vi "04TRM800.vi"() -> ()   [LabVIEW 2015]
uses:
  <vilib>/Utility/error.llb/DialogType.ctl
  <vilib>/Instr/_visa.llb/VISA Configure Serial Port (Serial Instr).vi
panel:
  out "Messages":string
  in  "INC":dbl min=-3.0 max=15.0 step=0.5 format="%.1g"
  in  "stop":bool
  out "String":string
  in  "LPCA COM Port":refnum<visa-resource-name>
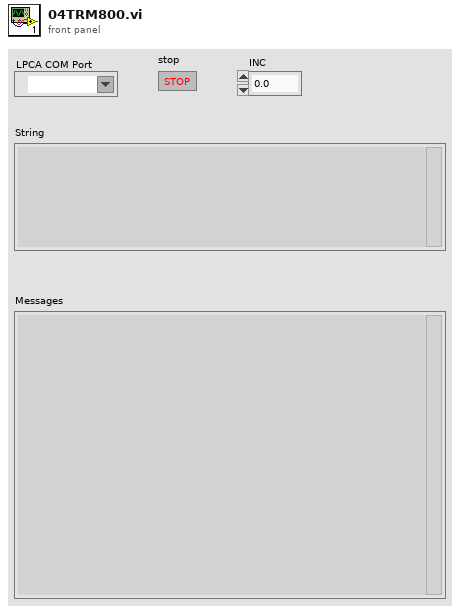
[diagram p1: front panel]
types:
  T1 = enum16{"Initialize", "Error", "Close", "Next", "Send"}
  T2 = enum16{"Initialize", "Next", "SendRSET", "SetMPH", "SetINC"}
  T3 = typedef "DialogType.ctl" = u16
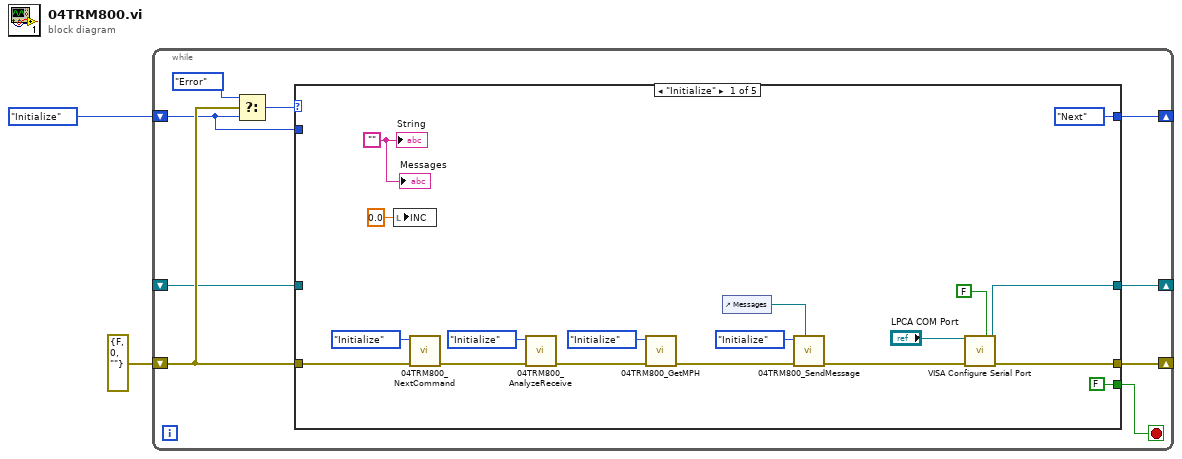
[diagram p0: block diagram]
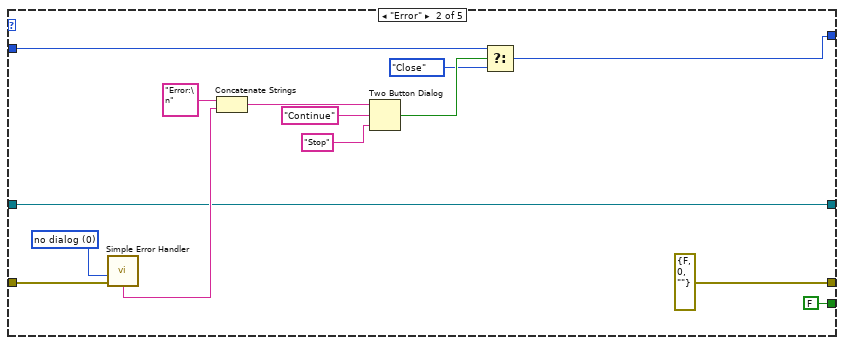
[diagram p2: hidden frame]
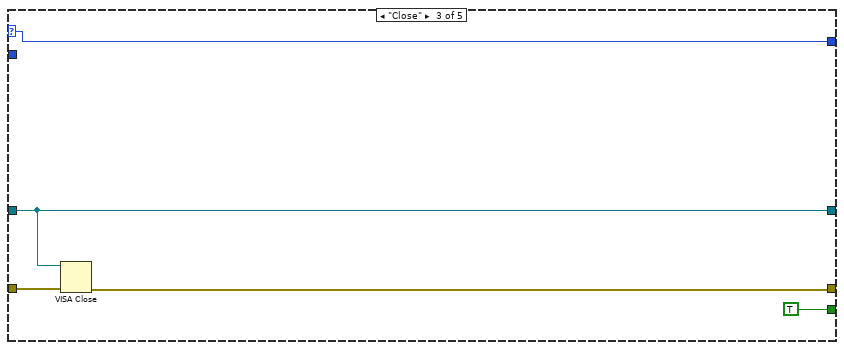
[diagram p3: hidden frame]
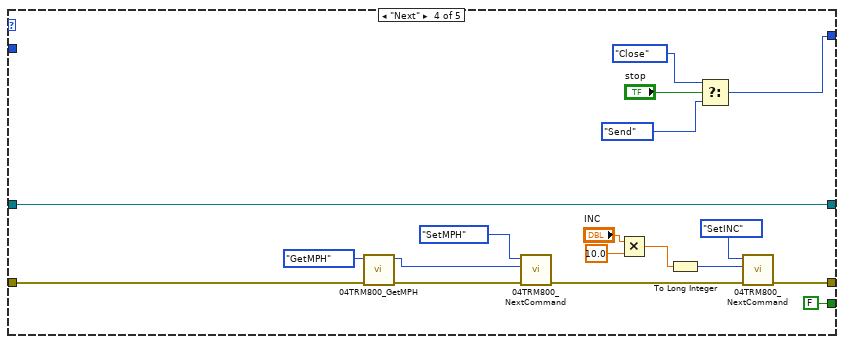
[diagram p4: hidden frame]
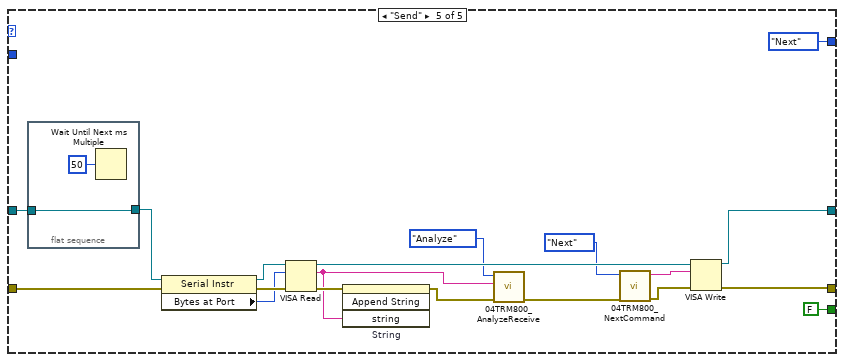
[diagram p5: hidden frame]
diagram:
  n1 = while {
    shift-right: [w9] -> _
    shift-left: T1."Initialize" -> [w8]
    shift-right: [w7] -> _
    shift-left: errorcluster {"status"=FALSE, "code"=0, "source"=""} ("error constant") -> [w11]
    shift-right: [w6] -> _
    shift-left: _ -> [w5]
    stop <- w4 stop-if-true
    n2 = Select(t=T1."Error", s=w11, f=w8) -> (s? t:f=w10:T1)
    n3 = case shown="\"Initialize\"" w10 {
      selector: w10 -> [_ _ w48 _ _]
      tunnel: w11 -> [w23 w43 w47 w52 w83]
      tunnel: [T1."Next" ("t") w33 w48 w61 T1."Next" ("t")] -> w9
      tunnel: w8 -> [_ w35 _ _ _]
      tunnel: [w29 errorcluster {"status"=FALSE, "code"=0, "source"=""} ("error constant") w45 w60 w73] -> w7
      tunnel: [w28 w32 w46 w65 w72] -> w6
      tunnel: w5 -> [_ w32 w46 w65 w84]
      tunnel: [FALSE FALSE TRUE FALSE FALSE] -> w4
      frame "Initialize" {
        w16 = ""
        n4 = local write "INC"(0.0 ("INC")) -> ()
        n5 = call "04TRM800_NextCommand.vi"("error in (no error)"=w23, "Enum"=enum16{"Initialize", "Next", "SendRSET"}."Initialize") -> ("error out"=w21:errorcluster)  [unwired: 8 in, 1 out]
        n6 = call "04TRM800_AnalyzeReceive.vi"("error in (no error)"=w21, "Enum"=enum16{"Initialize", "Analyze"}."Initialize") -> ("error out"=w18:errorcluster)  [unwired: 9 in]
        n7 = call "04TRM800_GetMPH.vi"("error in (no error)"=w18, "Initialize"=enum16{"Initialize", "GetMPH"}."Initialize") -> ("error out"=w15:errorcluster)  [unwired: 8 in, 1 out]
        n8 = control-ref of="Messages"() -> (w12:refnum<vi>)
        n9 = call "04TRM800_SendMessage.vi"("Str Refnum"=w12, "error in (no error)"=w15, "Enum"=enum16{"Initialize", "Send Message"}."Initialize") -> ("error out"=w14:errorcluster)  [unwired: 8 in]
        n10 = call-poly "VISA Configure Serial Port"("VISA resource name"="LPCA COM Port", "Enable Termination\nChar (T)"=FALSE ("Enable Termination\nChar (T)"), "error in (no error)"=w14) -> ("VISA resource name out"=w28:refnum<visa-resource-name>, "error out"=w29:errorcluster)  [unwired: 11 in]
        "String" <- w16
        "Messages" <- w16
      }
      frame "Error" {
        w30 = T3 0 items=["no dialog", "OK message", "continue or stop message", "OK message + warnings", "continue/stop + warnings"] ("type of dialog (OK msg:1)")
        n11 = call <vilib>:"Simple Error Handler.vi"("type of dialog (OK msg:1)"=w30, "error in (no error)"=w43) -> ("message"=w40:string)  [unwired: 3 in, 4 out]
        n12 = Concatenate Strings("Error:\n" ("string"), w40) -> (w41:string)
        n13 = Two Button Dialog(message=w41, 1:"Stop" ("F button name (\"Cancel\")"), 2:"Continue" ("T button name (\"OK\")")) -> (T button?=w36:bool)
        n14 = Select(t=w35, s=w36, f=enum16{"Initialize", "Error", "Close"}."Close") -> (s? t:f=w33:T1)
      }
      frame "Close" {
        n15 = VISA Close(VISA resource name=w46, error in (no error)=w47) -> (error out=w45:errorcluster)
      }
      frame "Next" {
        n16 = call "04TRM800_GetMPH.vi"("error in (no error)"=w52, "Initialize"=enum16{"Initialize", "GetMPH"}."GetMPH") -> ("error out"=w51:errorcluster, "MPH"=w50:i32)  [unwired: 8 in]
        n17 = call "04TRM800_NextCommand.vi"("error in (no error)"=w51, "Value"=w50, "Enum"=T2."SetMPH") -> ("error out"=w58:errorcluster)  [unwired: 7 in, 1 out]
        n18 = Multiply(x="INC", y=10.0) -> (x*y=w54:dbl)
        n19 = To Long Integer(number=w54) -> (32bit integer=w53:i32)
        n20 = Select(t=T1."Close", s="stop", f=T1."Send" ("t")) -> (s? t:f=w61:T1)
        n21 = call "04TRM800_NextCommand.vi"("error in (no error)"=w58, "Value"=w53, "Enum"=T2."SetINC") -> ("error out"=w60:errorcluster)  [unwired: 7 in, 1 out]
      }
      frame "Send" {
        n22 = flat-sequence {
          tunnel: [w86] -> w82
          tunnel: w84 -> [w86]
          frame #0 {
            n23 = Wait Until Next ms Multiple(millisecond multiple=u32 50) -> ()  [unwired: 1 out]
          }
        }
        n24 = property class="Serial Instr"(reference=w82, error in=w83) -> (reference out=w80:refnum<visa-resource-name>, error out=w81:errorcluster, "Bytes at Port"=w79:u32)
        n25 = VISA Read(VISA resource name=w80, byte count=w79, error in (no error)=w81) -> (VISA resource name out=w75:refnum<visa-resource-name>, read buffer=w71:string, error out=w78:errorcluster)  [unwired: 1 out]
        n26 = invoke on="String" class="Str" method="Append String"(error in=w78, "string"=w71) -> (error out=w70:errorcluster)  [unwired: 2 in, 3 out]
        n27 = call "04TRM800_AnalyzeReceive.vi"("error in (no error)"=w70, "String"=w71, "Enum"=enum16{"Initialize", "Analyze"}."Analyze") -> ("error out"=w69:errorcluster)  [unwired: 8 in]
        n28 = call "04TRM800_NextCommand.vi"("error in (no error)"=w69, "Enum"=T2."Next") -> ("error out"=w74:errorcluster, "String"=w76:string)  [unwired: 8 in]
        n29 = VISA Write(VISA resource name=w75, write buffer=w76, error in (no error)=w74) -> (VISA resource name out=w72:refnum<visa-resource-name>, error out=w73:errorcluster)  [unwired: 1 out]
      }
    }
  }
